vi "getEiting.vi"(8 "error in (no error)":errorcluster, 11 "ActionPanel.lvclass in":refnum<class "ActionPanel.lvclass">) -> (0 "error out":errorcluster, 2 "editing?":bool, 3 "ActionPanel.lvclass out":refnum<class "ActionPanel.lvclass">)   [LabVIEW 2011, in "Views.lvlib" / "ScriptEditor.lvlib" / "ActionPanel.lvclass"]
uses:
  ActionPanel.lvclass
  ActionPanel.lvclass/ActionPanel.ctl
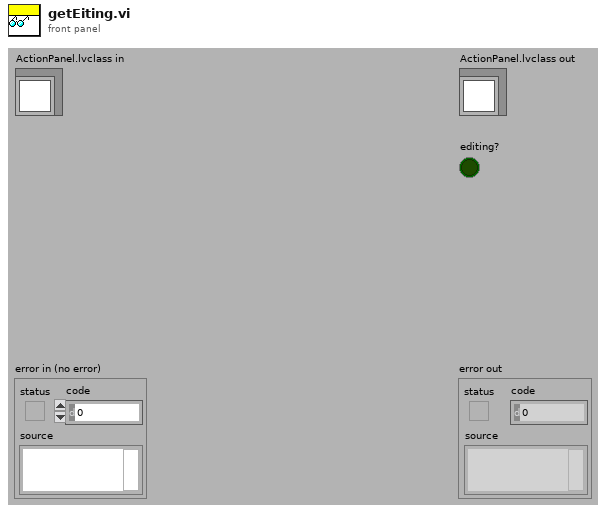
[diagram p1: front panel]
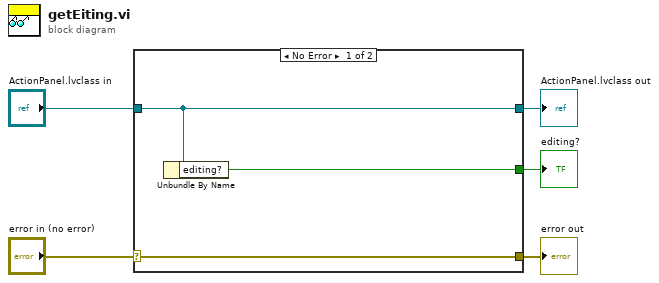
[diagram p0: block diagram]
diagram:
  n1 = case shown="No Error" "error in (no error)" {
    selector: "error in (no error)" -> [w8 w9]
    tunnel: [w8 w9] -> w4
    tunnel: [w7 w10] -> w2
    tunnel: "ActionPanel.lvclass in" -> [w7 w10]
    tunnel: [w6 _] -> w1
    frame No Error {
      n2 = Unbundle By Name(w7) -> ("editing?"=w6:bool)
    }
    frame Error {
    }
  }
  "error out" <- w4
  "ActionPanel.lvclass out" <- w2
  "editing?" <- w1
